vi "create camera controller.vi"(8 "error in (no error)":errorcluster, 11 "Camera Driver.lvclass":refnum<class "Camera Driver.lvclass">) -> (0 "error out":errorcluster, 3 "Camera Controller out":refnum<class "Camera Controller.lvclass">)   [LabVIEW 2022 SP3, in "Camera Controller.lvclass"]
uses:
  Camera Controller.lvclass
  Camera Driver/Camera Driver.lvclass
  Camera Controller.lvclass/Camera Controller.ctl
  Camera Process/Camera Process.lvclass
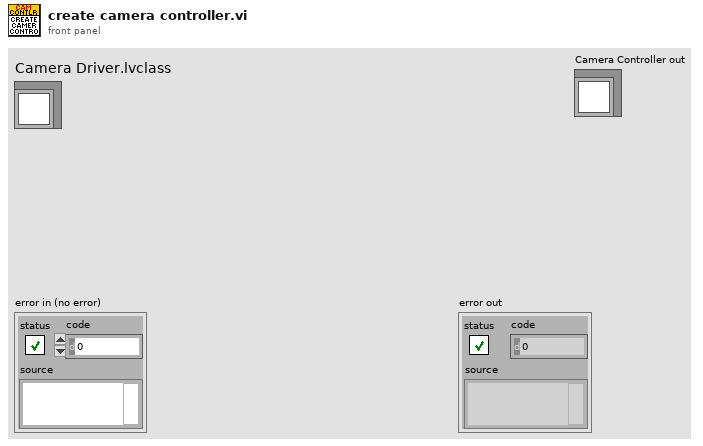
[diagram p1: front panel]
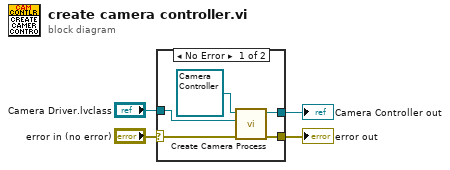
[diagram p0: block diagram]
diagram:
  n1 = case shown="No Error" "error in (no error)" {
    selector: "error in (no error)" -> [w6 w10]
    tunnel: [w5 w10] -> w3
    tunnel: [w8 _] -> w2
    tunnel: "Camera Driver.lvclass" -> [w7 _]
    frame No Error {
      n2 = call "Create Camera Process.vi"("error in (no error)"=w6, "Camera Driver.lvclass"=w7, "Camera Controller in"=refnum<class "Camera Controller.lvclass"> refnum) -> ("error out"=w5:errorcluster, "Camera Controller"=w8:refnum<class "Camera Controller.lvclass">)  [unwired: 7 in]
    }
    frame Error {
    }
  }
  "error out" <- w3
  "Camera Controller out" <- w2
